vi "Set Digital Pulls.vi"(8 "error in (no error)":errorcluster, 9 "Pull":T1, 10 "Channel":i32, 11 "VISA resource name in":refnum<visa-resource-name>) -> (0 "error out":errorcluster, 3 "VISA resource name":refnum<visa-resource-name>)   [LabVIEW 2020, in "CTI-Visa.lvlib"]
uses:
  CTI-Visa.lvlib
  Digital Pull Direction.ctl
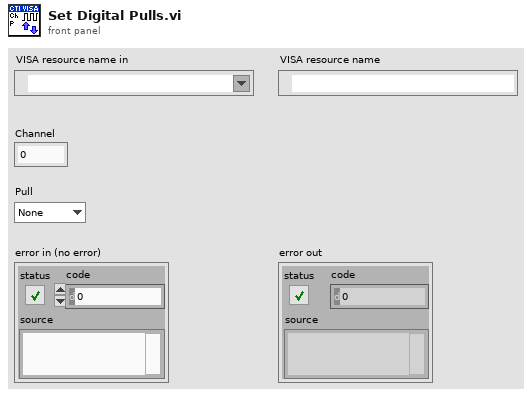
[diagram p1: front panel]
types:
  T1 = typedef "CTI-Visa.lvlib/Digital Pull Direction.ctl" = enum16{"None", "Up", "Down", "Both"}
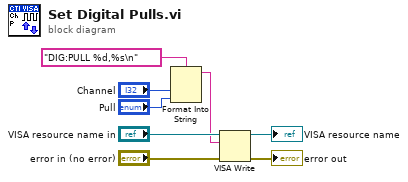
[diagram p0: block diagram]
diagram:
  n1 = Format Into String(format string="DIG:PULL %d,%s\n", "Channel", "Pull") -> (resulting string=w3:string)  [unwired: 2 in, 1 out]
  n2 = VISA Write(VISA resource name="VISA resource name in", write buffer=w3, error in (no error)="error in (no error)") -> (VISA resource name out=→"VISA resource name":refnum<visa-resource-name>, error out=→"error out":errorcluster)  [unwired: 1 out]
